vi "Convert from JSON Comp Format.vi"(8 "error in (no error)":errorcluster, 11 "JSON format":T6) -> (0 "error out":errorcluster, 3 "digital audio protocol settings":T1={"number of channels"=0, "data justification"=enum."Left Justified", "endianness"=enum."LSB First", "channel length"=0, "bit depth"=0, "frame clock rate"=0.0, "bit clock edge sync"=enum."Falling", "master clock rate"=0.0, "Logic Level"=enum."1.2 V", "frame sync edge for channel 0"=enum."Rising", "Channel 0 Offset"=0})   [LabVIEW 2023, in "digital audio protocol controls.lvlib"]
uses:
  digital audio protocol controls.lvlib
  digital serial gen settings_json.ctl
  controls/digital serial gen settings.ctl
  <vilib>/PDM Acquisition Toolkit/shared/controls/PCM Data Justification.ctl
  <vilib>/PDM Acquisition Toolkit/shared/controls/PCM Bit Endianness.ctl
  <vilib>/PDM Acquisition Toolkit/shared/controls/Digital Edge.ctl
  <vilib>/PDM Acquisition Toolkit/host/Classes/Session/Controls/Logic Levels.ctl
  <vilib>/PDM Acquisition Toolkit/shared/PDM Shared.lvlib
  <vilib>/PDM Acquisition Toolkit/host/Classes/Session/DecoderSession.lvclass
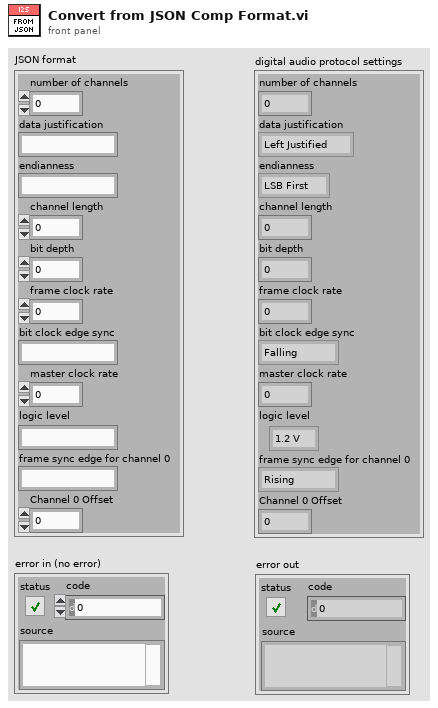
[diagram p1: front panel]
types:
  T1 = typedef "digital serial gen settings.ctl" = cluster{"number of channels":u32, "data justification":T2, "endianness":T3, "channel length":u32, "bit depth":u32, "frame clock rate":dbl, "bit clock edge sync":T4, "master clock rate":dbl, "Logic Level":T5, "frame sync edge for channel 0":T4, "Channel 0 Offset":u32}
  T2 = typedef "PDM Shared.lvlib/PCM Data Justification.ctl" = enum16{"Left Justified", "Right Justified"}
  T3 = typedef "PDM Shared.lvlib/PCM Bit Endianness.ctl" = enum16{"MSB First", "LSB First"}
  T4 = typedef "PDM Shared.lvlib/Digital Edge.ctl" = enum8{"Rising", "Falling"}
  T5 = typedef "PDM Acquisition Class Library.lvlib/DecoderSession.lvclass/Logic Levels.ctl" = enum16{"3.3 V", "1.8 V", "1.2 V"}
  T6 = typedef "digital audio protocol controls.lvlib/digital serial gen settings_json.ctl" = cluster{"number of channels":u32, "data justification":string, "endianness":string, "channel length":u32, "bit depth":u32, "frame clock rate":dbl, "bit clock edge sync":string, "master clock rate":dbl, "logic level":string, "frame sync edge for channel 0":string, "Channel 0 Offset":u32}
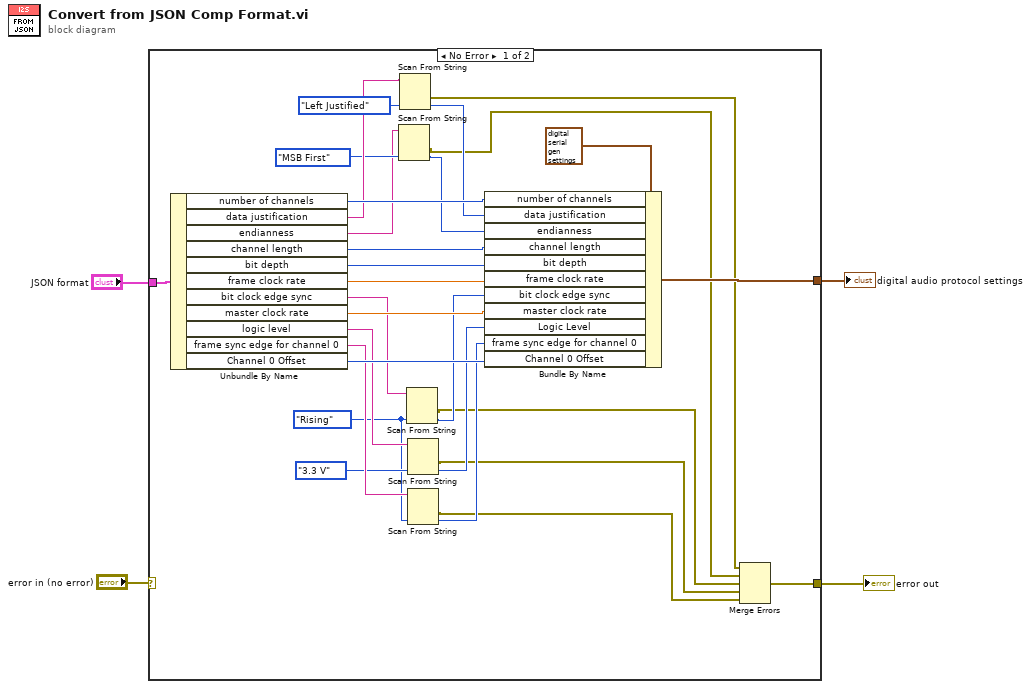
[diagram p0: block diagram]
diagram:
  n1 = case shown="No Error" "error in (no error)" {
    selector: "error in (no error)" -> [_ w34]
    tunnel: "JSON format" -> [w26 _]
    tunnel: [w25 _] -> w3
    tunnel: [w5 w34] -> w1
    frame No Error {
      w14 = Digital_Edge."Rising" ("bit clock edge sync")
      n2 = Unbundle By Name(w26) -> ("number of channels"=w33:u32, "data justification"=w24:string, "endianness"=w20:string, "channel length"=w32:u32, "bit depth"=w31:u32, "frame clock rate"=w30:dbl, "bit clock edge sync"=w18:string, "master clock rate"=w29:dbl, "logic level"=w17:string, "frame sync edge for channel 0"=w16:string, "Channel 0 Offset"=w28:u32)
      n3 = Scan From String(input string=w20, default 1=PCM_Bit_Endianness."MSB First" ("endianness")) -> (error out=w9:errorcluster, output 1=w19:T3)  [unwired: 3 in, 2 out]
      n4 = Scan From String(input string=w24, default 1=PCM_Data_Justification."Left Justified" ("data justification")) -> (error out=w10:errorcluster, output 1=w22:T2)  [unwired: 3 in, 2 out]
      n5 = Scan From String(input string=w18, default 1=w14) -> (error out=w8:errorcluster, output 1=w13:T4)  [unwired: 3 in, 2 out]
      n6 = Scan From String(input string=w17, default 1=Logic_Levels."3.3 V" ("Logic Level")) -> (error out=w7:errorcluster, output 1=w12:T5)  [unwired: 3 in, 2 out]
      n7 = Scan From String(input string=w16, default 1=w14) -> (error out=w6:errorcluster, output 1=w11:T4)  [unwired: 3 in, 2 out]
      n8 = Bundle By Name(cluster=T1 {"number of channels"=0, "data justification"=enum."Left Justified", "endianness"=enum."LSB First", "channel length"=0, "bit depth"=0, "frame clock rate"=0.0, "bit clock edge sync"=enum."Falling", "master clock rate"=0.0, "Logic Level"=enum."1.2 V", "frame sync edge for channel 0"=enum."Rising", "Channel 0 Offset"=0} ("digital audio protocol settings"), "number of channels"=w33, "data justification"=w22, "endianness"=w19, "channel length"=w32, "bit depth"=w31, "frame clock rate"=w30, "bit clock edge sync"=w13, "master clock rate"=w29, "Logic Level"=w12, "frame sync edge for channel 0"=w11, "Channel 0 Offset"=w28) -> (w25:T1)
      n9 = Merge Errors(w10, w9, w8, w7, w6) -> (w5:errorcluster)
    }
    frame Error {
    }
  }
  "digital audio protocol settings" <- w3
  "error out" <- w1
